vi "_start_measure.vi"(8 "error in (no error)":errorcluster, 9 "a_Nmsr":i16, 10 "a_hWnd":i32, 11 "UV-VIS_AVANTES in":refnum<class "UV-VIS_AVANTES.lvclass">) -> (0 "error out":errorcluster, 3 "UV-VIS_AVANTES out":refnum<class "UV-VIS_AVANTES.lvclass">)   [LabVIEW 2020, in "UV-VIS_AVANTES.lvclass"]
uses:
  UV-VIS_AVANTES.lvclass
  C:/Dev/TRANCON/Classes/Detector/Detector.lvclass
  Detector.lvclass/Detector.ctl
  UV-VIS_AVANTES.lvclass/UV-VIS_AVANTES.ctl
  Detector.lvclass
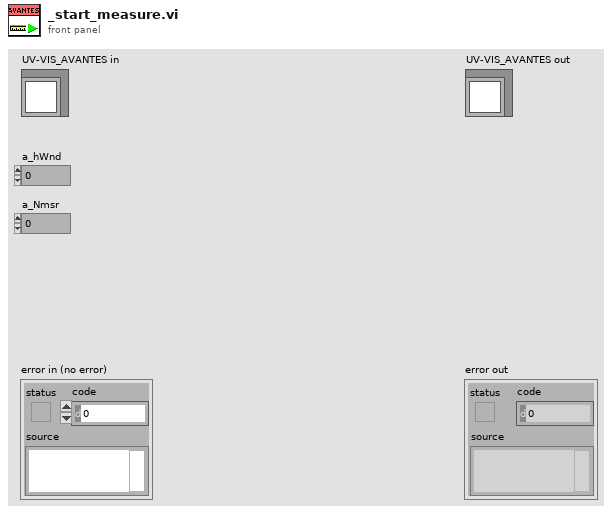
[diagram p1: front panel]
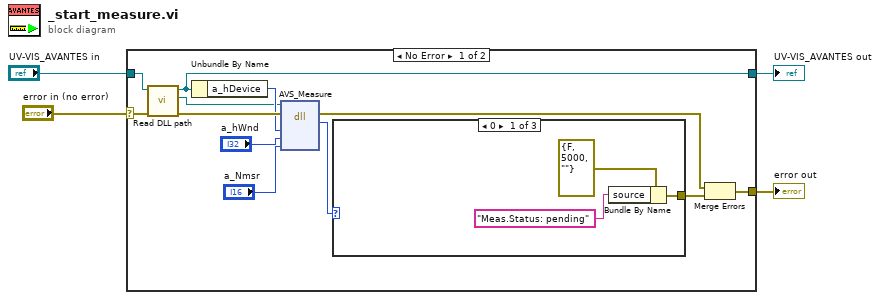
[diagram p0: block diagram]
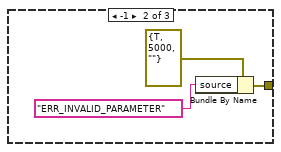
[diagram p2: hidden frame]
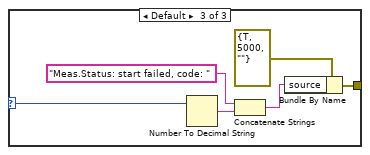
[diagram p3: hidden frame]
diagram:
  n1 = case shown="No Error" "error in (no error)" {
    selector: "error in (no error)" -> [w15 w30]
    tunnel: [w5 w30] -> w3
    tunnel: [w14 w29] -> w1
    tunnel: "UV-VIS_AVANTES in" -> [w16 w29]
    frame No Error {
      n2 = call "Read DLL path.vi"("error in (no error)"=w15, "Detector in"=w16) -> ("error out"=w11:errorcluster, "DLL path"=w9:path, "Detector out"=w14:refnum<class "UV-VIS_AVANTES.lvclass">)  [unwired: 7 in]
      n3 = Unbundle By Name(w14) -> ("a_hDevice"=w10:i32)
      n4 = dll-call lib="C:/AvaSpecX64-DLL_9.4/examples/LabView/LabViewSingleChan/avaspec.dll" fn="AVS_Measure"(path in=w9, error in=w11, "a_hDevice"=w10, "a_hWnd"="a_hWnd", "a_Nmsr"="a_Nmsr") -> (error out=w7:errorcluster, "return type"=w8:i32)  [unwired: 4 in, 1 out]
      n5 = case shown="0" w8 {
        selector: w8 -> [_ _ w28]
        tunnel: [w17 w20 w24] -> w6
        frame 0 {
          n6 = Bundle By Name(cluster=errorcluster {"status"=FALSE, "code"=5000, "source"=""} ("error out"), "source"="Meas.Status: pending") -> (w17:errorcluster)
        }
        frame -1 {
          n7 = Bundle By Name(cluster=errorcluster {"status"=TRUE, "code"=5000, "source"=""} ("error out"), "source"="ERR_INVALID_PARAMETER") -> (w20:errorcluster)
        }
        frame Default {
          n8 = Number To Decimal String(number=w28) -> (decimal integer string=w27:string)  [unwired: 1 in]
          n9 = Concatenate Strings("Meas.Status: start failed, code: ", w27) -> (w23:string)
          n10 = Bundle By Name(cluster=errorcluster {"status"=TRUE, "code"=5000, "source"=""} ("error out"), "source"=w23) -> (w24:errorcluster)
        }
      }
      n11 = Merge Errors(w7, w6) -> (w5:errorcluster)
    }
    frame Error {
    }
  }
  "error out" <- w3
  "UV-VIS_AVANTES out" <- w1
